vi "NETCallback FileWatcher Simple.vi"(4 "queue out":refnum<queue>, 5 "Event Data":cluster{"sender":refnum<k24>, "e":refnum<k24>}, 6 "Control Ref":refnum<k24>, 7 "Event Common Data":T1) -> ()   [LabVIEW 2021]
uses:
  <vilib>/JDP Science/JSONtext/LVClass Serializer/JSONtext LVClass Serializer.lvclass
  5b99c23a-5df9-4087-89f4-512f78e848ed.vi
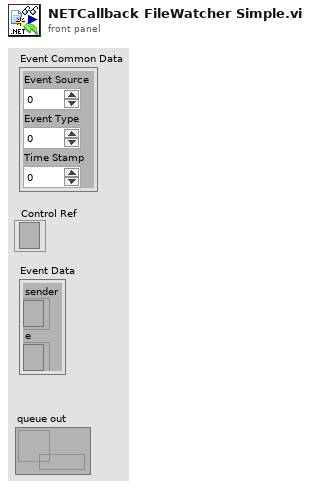
[diagram p1: front panel]
types:
  T1 = cluster{"Event Source":i32, "Event Type":u32, "Time Stamp":u32}
  T2 = cluster{"ToString":string, "ChangeType":i32, "FullPath":string, "Name":string}
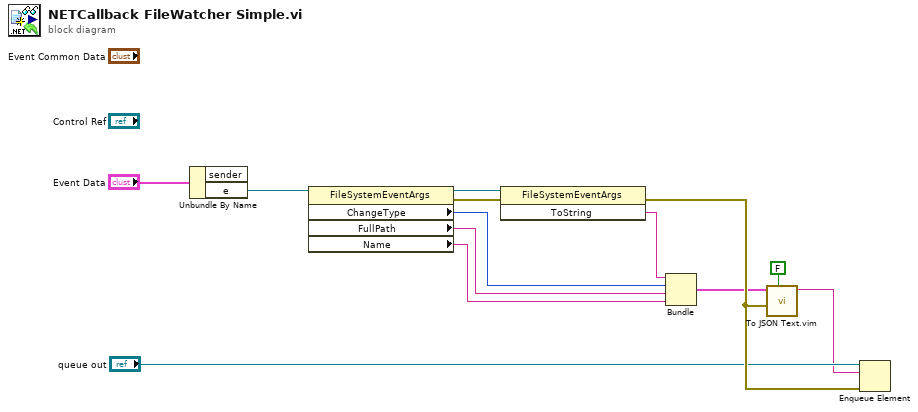
[diagram p0: block diagram]
diagram:
  n1 = Unbundle By Name("Event Data") -> ("e"=w11:refnum<k24>)  [unwired: 1 out]
  n2 = property class="FileSystemEventArgs"(reference=w11) -> (reference out=w10:refnum<k24>, error out=w2:errorcluster, "ChangeType"=w8:i32, "FullPath"=w7:string, "Name"=w6:string)  [unwired: 1 in]
  n3 = invoke class="FileSystemEventArgs" method="ToString"(reference=w10, error in=w2) -> (error out=w13:errorcluster, "ToString"=w9:string)  [unwired: 1 in, 1 out]
  n4 = Bundle("ToString"=w9, "ChangeType"=w8, "FullPath"=w7, "Name"=w6) -> (w4:T2)  [unwired: 1 in]
  n5 = call "To JSON Text.vim"("enable LabVIEW extensions? (T)"=FALSE, "error in (no error)"=w13, "Anything"=w4) -> ("<JSON>"=w3:string)  [unwired: 7 in, 1 out]
  n6 = Enqueue Element(queue="queue out", element=w3, error in (no error)=w13) -> ()  [unwired: 1 in, 3 out]
